vi "Traverse for BD Refs.vi"(8 "error in (no error)":errorcluster, 9 "GObject Ref":refnum<vi>, 11 "Refs in":T1) -> (0 "error out":errorcluster, 1 "Stop Traverse":bool, 3 "Refs":T1)   [LabVIEW 2020, in "FlexBlocks.lvlib"]
uses:
  FlexBlocks.lvlib
  Scripting Refs.ctl
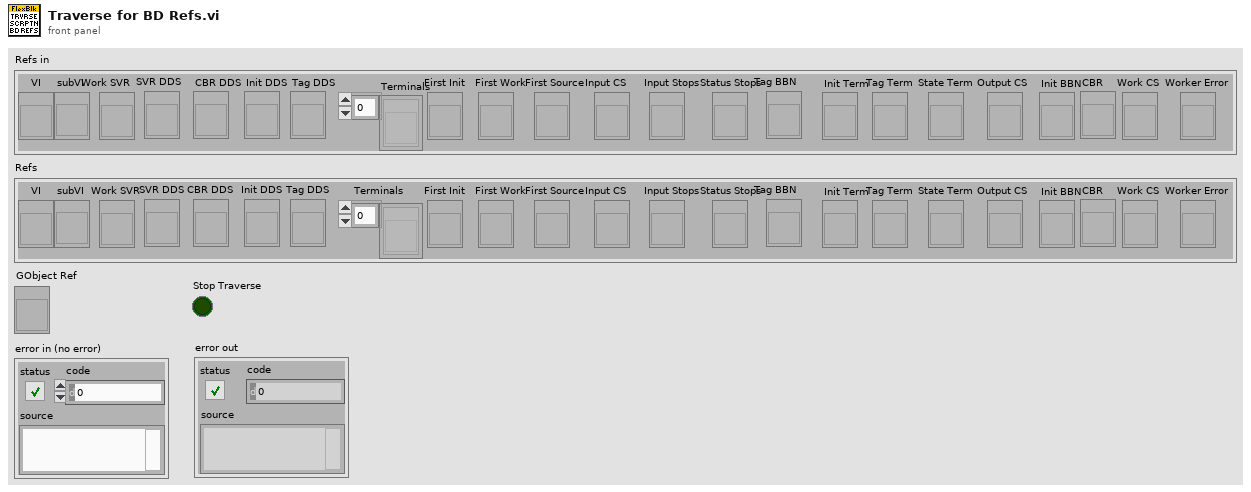
[diagram p1: front panel]
types:
  T1 = typedef "FlexBlocks.lvlib/Scripting Refs.ctl" = cluster{"VI":refnum<vi>, "subVI":refnum<vi>, "Work SVR":refnum<vi>, "SVR DDS":refnum<vi>, "CBR DDS":refnum<vi>, "Init DDS":refnum<vi>, "Tag DDS":refnum<vi>, "Terminals":refnum<vi>[], "First Init":refnum<vi>, "First Work":refnum<vi>, "First Source":refnum<vi>, "Input CS":refnum<vi>, "Input Stops":refnum<vi>, "Status Stops":refnum<vi>, "Tag BBN":refnum<vi>, "Init Term":refnum<vi>, "Tag Term":refnum<vi>, "State Term":refnum<vi>, "Output CS":refnum<vi>, "Init BBN":refnum<vi>, "CBR":refnum<vi>, "Work CS":refnum<vi>, "Worker Error":refnum<vi>}
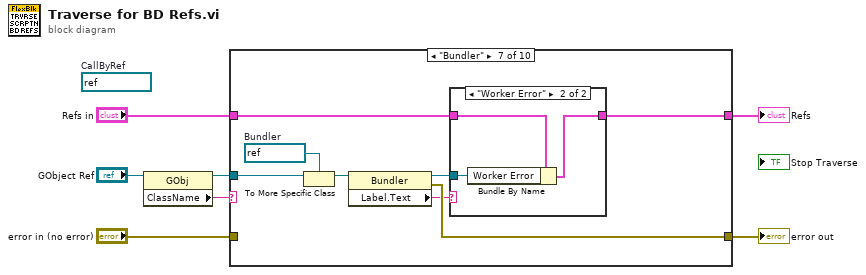
[diagram p0: block diagram]
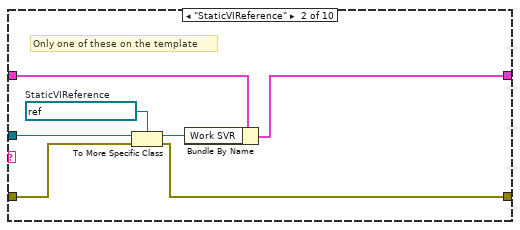
[diagram p3: hidden frame]
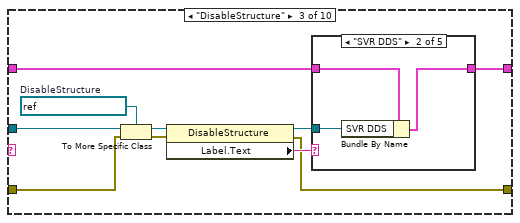
[diagram p4: hidden frame]
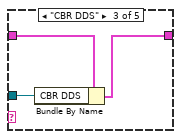
[diagram p6: hidden frame]
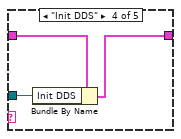
[diagram p7: hidden frame]
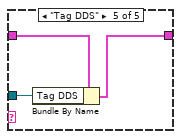
[diagram p8: hidden frame]
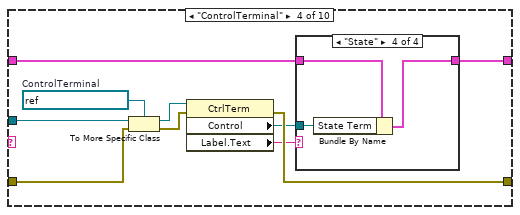
[diagram p9: hidden frame]
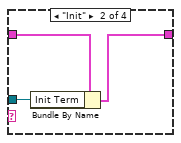
[diagram p11: hidden frame]
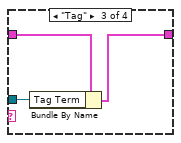
[diagram p12: hidden frame]
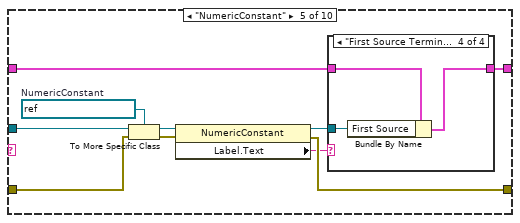
[diagram p13: hidden frame]
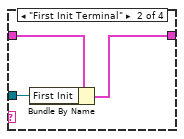
[diagram p15: hidden frame]
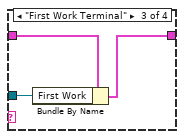
[diagram p16: hidden frame]
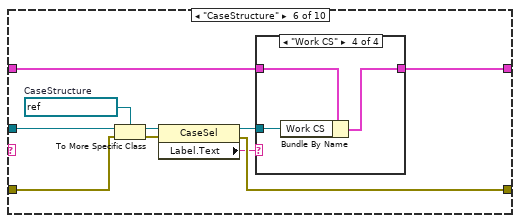
[diagram p17: hidden frame]
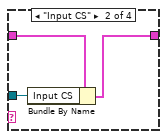
[diagram p19: hidden frame]
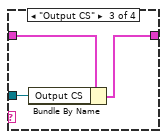
[diagram p20: hidden frame]
diagram:
  (unwired) refnum<vi> refnum  # CallByRef
  n1 = property class="GObj"(reference="GObject Ref") -> (reference out=w3:refnum<vi>, "ClassName"=w4:string)  [unwired: 1 in, 1 out]
  n2 = case shown="\"Bundler\"" w4 {
    tunnel: "error in (no error)" -> [w8 w11 w24 w47 w66 w87 _ w116 w126 w142]
    tunnel: "Refs in" -> [w9 w14 w19 w43 w61 w82 w101 w115 w121 w137]
    tunnel: w3 -> [_ w16 w26 w49 w68 w89 w106 w118 w128 w144]
    tunnel: [w9 w12 w18 w40 w60 w80 w100 w113 w120 w136] -> w2
    tunnel: [w8 w10 w17 w44 w69 w84 w107 w112 w122 w145] -> w1
    frame Default {
    }
    frame "StaticVIReference" {
      w15 = refnum<vi> refnum  # StaticVIReference
      # "Only one of these on the template"
      n3 = To More Specific Class(target class=w15, reference=w16, error in=w11) -> (specific class reference=w13:refnum<vi>, error out=w10:errorcluster)
      n4 = Bundle By Name(cluster=w14, "Work SVR"=w13) -> (w12:T1)
    }
    frame "DisableStructure" {
      w25 = refnum<vi> refnum  # DisableStructure
      n5 = To More Specific Class(target class=w25, reference=w26, error in=w24) -> (specific class reference=w23:refnum<vi>, error out=w22:errorcluster)
      n6 = property class="DisableStructure"(reference=w23, error in=w22) -> (reference out=w20:refnum<vi>, error out=w17:errorcluster, "Label.Text"=w21:string)
      n7 = case shown="\"SVR DDS\"" w21 {
        tunnel: w20 -> [_ w29 w32 w35 w38]
        tunnel: w19 -> [w27 w30 w33 w36 w39]
        tunnel: [w27 w28 w31 w34 w37] -> w18
        frame Default {
        }
        frame "SVR DDS" {
          n8 = Bundle By Name(cluster=w30, "SVR DDS"=w29) -> (w28:T1)
        }
        frame "CBR DDS" {
          n9 = Bundle By Name(cluster=w33, "CBR DDS"=w32) -> (w31:T1)
        }
        frame "Init DDS" {
          n10 = Bundle By Name(cluster=w36, "Init DDS"=w35) -> (w34:T1)
        }
        frame "Tag DDS" {
          n11 = Bundle By Name(cluster=w39, "Tag DDS"=w38) -> (w37:T1)
        }
      }
    }
    frame "ControlTerminal" {
      w48 = refnum<vi> refnum  # ControlTerminal
      n12 = To More Specific Class(target class=w48, reference=w49, error in=w47) -> (specific class reference=w46:refnum<vi>, error out=w45:errorcluster)
      n13 = property class="CtrlTerm"(reference=w46, error in=w45) -> (error out=w44:errorcluster, "Control"=w41:refnum<vi>, "Label.Text"=w42:string)  [unwired: 1 out]
      n14 = case shown="\"State\"" w42 {
        tunnel: w43 -> [w50 w53 w56 w59]
        tunnel: w41 -> [_ w52 w55 w58]
        tunnel: [w50 w51 w54 w57] -> w40
        frame Default {
        }
        frame "Init" {
          n15 = Bundle By Name(cluster=w53, "Init Term"=w52) -> (w51:T1)
        }
        frame "Tag" {
          n16 = Bundle By Name(cluster=w56, "Tag Term"=w55) -> (w54:T1)
        }
        frame "State" {
          n17 = Bundle By Name(cluster=w59, "State Term"=w58) -> (w57:T1)
        }
      }
    }
    frame "NumericConstant" {
      w67 = refnum<vi> refnum  # NumericConstant
      n18 = To More Specific Class(target class=w67, reference=w68, error in=w66) -> (specific class reference=w65:refnum<vi>, error out=w64:errorcluster)
      n19 = property class="NumericConstant"(reference=w65, error in=w64) -> (reference out=w63:refnum<vi>, error out=w69:errorcluster, "Label.Text"=w62:string)
      n20 = case shown="\"First Source Terminal\"" w62 {
        tunnel: w63 -> [_ w72 w75 w78]
        tunnel: w61 -> [w70 w73 w76 w79]
        tunnel: [w70 w71 w74 w77] -> w60
        frame Default {
        }
        frame "First Init Terminal" {
          n21 = Bundle By Name(cluster=w73, "First Init"=w72) -> (w71:T1)
        }
        frame "First Work Terminal" {
          n22 = Bundle By Name(cluster=w76, "First Work"=w75) -> (w74:T1)
        }
        frame "First Source Terminal" {
          n23 = Bundle By Name(cluster=w79, "First Source"=w78) -> (w77:T1)
        }
      }
    }
    frame "CaseStructure" {
      w88 = refnum<vi> refnum  # CaseStructure
      n24 = To More Specific Class(target class=w88, reference=w89, error in=w87) -> (specific class reference=w86:refnum<vi>, error out=w85:errorcluster)
      n25 = property class="CaseSel"(reference=w86, error in=w85) -> (reference out=w81:refnum<vi>, error out=w84:errorcluster, "Label.Text"=w83:string)
      n26 = case shown="\"Work CS\"" w83 {
        tunnel: w82 -> [w90 w93 w96 w99]
        tunnel: w81 -> [_ w92 w95 w98]
        tunnel: [w90 w91 w94 w97] -> w80
        frame Default {
        }
        frame "Input CS" {
          n27 = Bundle By Name(cluster=w93, "Input CS"=w92) -> (w91:T1)
        }
        frame "Output CS" {
          n28 = Bundle By Name(cluster=w96, "Output CS"=w95) -> (w94:T1)
        }
        frame "Work CS" {
          n29 = Bundle By Name(cluster=w99, "Work CS"=w98) -> (w97:T1)
        }
      }
    }
    frame "Bundler" {
      w105 = refnum<vi> refnum  # Bundler
      n30 = To More Specific Class(target class=w105, reference=w106) -> (specific class reference=w104:refnum<vi>)  [unwired: 1 in, 1 out]
      n31 = property class="Bundler"(reference=w104) -> (reference out=w102:refnum<vi>, error out=w107:errorcluster, "Label.Text"=w103:string)  [unwired: 1 in]
      n32 = case shown="\"Worker Error\"" w103 {
        tunnel: w102 -> [_ w110]
        tunnel: w101 -> [w108 w111]
        tunnel: [w108 w109] -> w100
        frame Default {
        }
        frame "Worker Error" {
          n33 = Bundle By Name(cluster=w111, "Worker Error"=w110) -> (w109:T1)
        }
      }
    }
    frame "CallByRef" {
      w117 = refnum<vi> refnum  # CallByRef
      # "Only one of these on the template"
      n34 = To More Specific Class(target class=w117, reference=w118, error in=w116) -> (specific class reference=w114:refnum<vi>, error out=w112:errorcluster)
      n35 = Bundle By Name(cluster=w115, "CBR"=w114) -> (w113:T1)
    }
    frame "CompoundArithmetic" {
      w127 = refnum<vi> refnum  # CompoundArithmetic
      n36 = To More Specific Class(target class=w127, reference=w128, error in=w126) -> (specific class reference=w125:refnum<vi>, error out=w124:errorcluster)
      n37 = property class="CmpArith"(reference=w125, error in=w124) -> (reference out=w119:refnum<vi>, error out=w122:errorcluster, "Label.Text"=w123:string)
      n38 = case shown="\"Status Stops\"" w123 {
        tunnel: w121 -> [w129 w132 w135]
        tunnel: [w129 w130 w133] -> w120
        tunnel: w119 -> [_ w131 w134]
        frame Default {
        }
        frame "Input Stops" {
          n39 = Bundle By Name(cluster=w132, "Input Stops"=w131) -> (w130:T1)
        }
        frame "Status Stops" {
          n40 = Bundle By Name(cluster=w135, "Status Stops"=w134) -> (w133:T1)
        }
      }
    }
    frame "NamedBundler" {
      w143 = refnum<vi> refnum  # NamedBundler
      n41 = To More Specific Class(target class=w143, reference=w144, error in=w142) -> (specific class reference=w141:refnum<vi>, error out=w140:errorcluster)
      n42 = property class="NmdBndl"(reference=w141, error in=w140) -> (reference out=w139:refnum<vi>, error out=w145:errorcluster, "Label.Text"=w138:string)
      n43 = case shown="\"Init BBN\"" w138 {
        tunnel: w139 -> [_ w148 w151]
        tunnel: w137 -> [w146 w149 w152]
        tunnel: [w146 w147 w150] -> w136
        frame Default {
        }
        frame "Tag BBN" {
          n44 = Bundle By Name(cluster=w149, "Tag BBN"=w148) -> (w147:T1)
        }
        frame "Init BBN" {
          n45 = Bundle By Name(cluster=w152, "Init BBN"=w151) -> (w150:T1)
        }
      }
    }
  }
  "error out" <- w1
  "Refs" <- w2
